vi "UI - FP and Controls.vi"(5 "Term (Methods)":string="Methods", 7 "Msg Chain":string, 8 "error in (no error)":errorcluster {"code" format="Error %.0f"}, 10 "UI Docs":refnum<class "GUI Documentation.lvclass">[](array[class]), 11 "VIDoc Printer - Confluence In":refnum<class "VIDoc Printer - Confluence.lvclass">) -> (0 "error out":errorcluster {"code" format="Error %.0f"}, 3 "VIDoc Printer - Confluence Out":refnum<class "VIDoc Printer - Confluence.lvclass">)   [LabVIEW 2023, in "VIDoc Printer - Confluence.lvlib" / "VIDoc Printer - Confluence.lvclass"]
uses:
  VIDoc Printer - Confluence.lvclass
  C:/projects/DMC/GitHub/DMC CLI VIDoc/Source/Documentation Generation/Printers/Printer/VIDoc Printer.lvclass
  Parsing/GUI Documentation/GUI Documentation.lvclass
  Printer/VIDoc Printer.lvclass/VIDoc Printer.ctl
  Parsing/GUI Documentation/GUI Documentation.lvclass/GUI Documentation.ctl
  VIDoc Printer - Confluence.lvclass/VIDoc Printer - Confluence.ctl
  Confluence Formatting/Types/Format Combo Box.ctl
  Types/VI Info Image Types.ctl
  81eb6c55-aa97-43e1-ad41-127c3d76b8c9.vi
  Printer/Accessors/Get VI Settings - Method Options - Front Panels.vi
  Printer/Accessors/Get VI Settings - Method Options - Options.vi
  Printer/Accessors/Get VI Settings - Method Options - Controls.vi
  Printer/Accessors/Get VI Settings - Controls Detail Level.vi
  Accessors/Get VI Controls Expand.vi
  Accessors/Get Sortable Tables.vi
  Parsing/GUI Documentation/Get VI Info.vi
  Parsing/GUI Documentation/Get Name.vi
  Confluence Formatting/Confluence Formatting.lvlib
  Printer/VIDoc Printer.lvclass
  UI Interaction/UI Interaction.lvclass
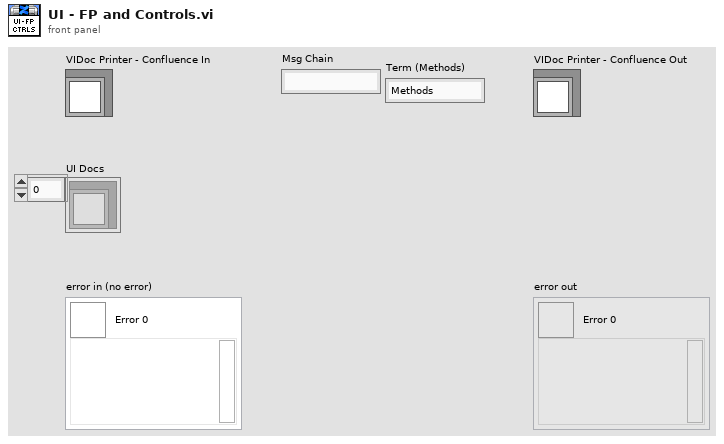
[diagram p1: front panel]
types:
  T1 = typedef "VIDoc Printer.lvlib/Printer Settings.lvclass/VI Settings.ctl" = cluster{"Memory":bool, "By Folder":bool, "By Tree":bool, "By List":bool, "Methods":bool, "Method Options":cluster{"Front Panels":bool, "Options":bool, "Controls":bool}, "List Detail Level":T2, "Methods Detail Level":T2, "Controls Detail Level":T2}
  T2 = typedef "VIDoc Printer.lvlib/Printer Settings.lvclass/Detail Level Enum.ctl" = enum16{"None", "Minimal", "Standard", "Full"}
  T3 = typedef "VIDoc Printer - Confluence.lvlib/VIDoc Printer - Confluence.lvclass/VI Info Image Types.ctl" = enum16{"Conpane", "FP", "BD", "Icon"}
  T4 = typedef "Confluence Formatting.lvlib/Format Combo Box.ctl" = string
  T5 = typedef "VIDoc Parsing.lvlib/Method Spec Cluster.ctl" = cluster{"VI Type Ext":T6, "Name":string, "Path":path, "Get Conpane Image":T7, "Description":string, "Get Library Access Scope":enum32{"invalid scope", "public", "private", "protected", "community"}, "Dispatch":T8, "ContainsCompiledCode":bool, "Exec.IsReentrant":bool, "Exec.ReentrancyType":enum16{"Share clones between instances", "Preallocate clone for each instance"}, "ExecInlining":bool, "ExecInlineIfPossible":bool, "Auto Err Handling":bool, "CodeComplexity":sgl, "Bookmark Tags":string[], "Control VI Type":enum32{"not a control VI", "control", "typedef", "strict typedef"}, "Controls":T9[], "VI Type":enum32{"invalid VI type", "Standard VI", "Control VI", "Global VI", "Polymorphic VI", "Configuration VI", "SubSystem", "Facade VI", "Method VI", "Statechart Diagram VI"}, "Minimum Size":T11, "Front Panel Window:Title":string, "Front Panel Window:Behavior":enum32{"Invalid", "Default", "Floating", "Floating/Auto-Hide", "Modal"}, "Front Panel Window:Closeable":bool, "Must Override":bool, "Must Use Parent Implementation":bool, "VI Icon":T7, "Front Panel":T7, "History:Revision Number":u32, "Metrics:Total Data Size":u32, "Execution:Allow Debugging":bool, "Execution:Preferred Exec System":enum32{"invalid execution system", "user interface", "standard", "instrument i/o", "data acquisition", "other 1", "other 2", "same as caller"}, "Execution:Priority":enum32{"invalid priority", "background priority", "normal priority", "above normal priority", "high priority", "time critical priority", "subroutine"}, "BM Tag Text":string[], "Block Diagram":T7, "Structure Tree":T12[]}
  T6 = typedef "VIDoc Parsing.lvlib/VI Type Extended Enum.ctl" = enum16{"Unknown", "Class Method", "Class Accessor Get", "Class Accessor Set", "Class Control", "Library Method", "Library Control", "VI", "Control"}
  T7 = typedef "imagedata.ctl" = cluster{"image type":i32, "image depth":i32, "image":u8[], "mask":u8[], "colors":u32[], "Rectangle":cluster{"left":i16, "top":i16, "right":i16, "bottom":i16}}
  T8 = typedef "VIDoc Parsing.lvlib/Class Dispatch Type Enum.ctl" = enum16{"None", "Static", "Dynamic"}
  T9 = typedef "VIDoc Parsing.lvlib/Controls Info Cluster.ctl" = cluster{"Name":string, "Description":string, "Data Type":string, "Tip Strip":string, "UID":i32, "Image Data":T7, "ToggleKeyBind":T10, "Raw Label":string, "Raw Caption":string}
  T10 = typedef "LVKeyTypeDef.ctl" = cluster{"Focus":bool, "Control":bool, "Shift":bool, "Key":string}
  T11 = typedef "LVPointTypeDef.ctl" = cluster{"Horizontal":i16, "Vertical":i16}
  T12 = typedef "VIDoc Parsing.lvlib/Structure Reporter.lvlib/Tree Cluster.ctl" = cluster{"Object Class Name":string, "Labels":string[], "Child Tag":string, "Item Indent":i32, "Child Only?":bool, "Glyph Index":i32}
  T13 = enum32{"not a control VI", "control", "typedef", "strict typedef"}
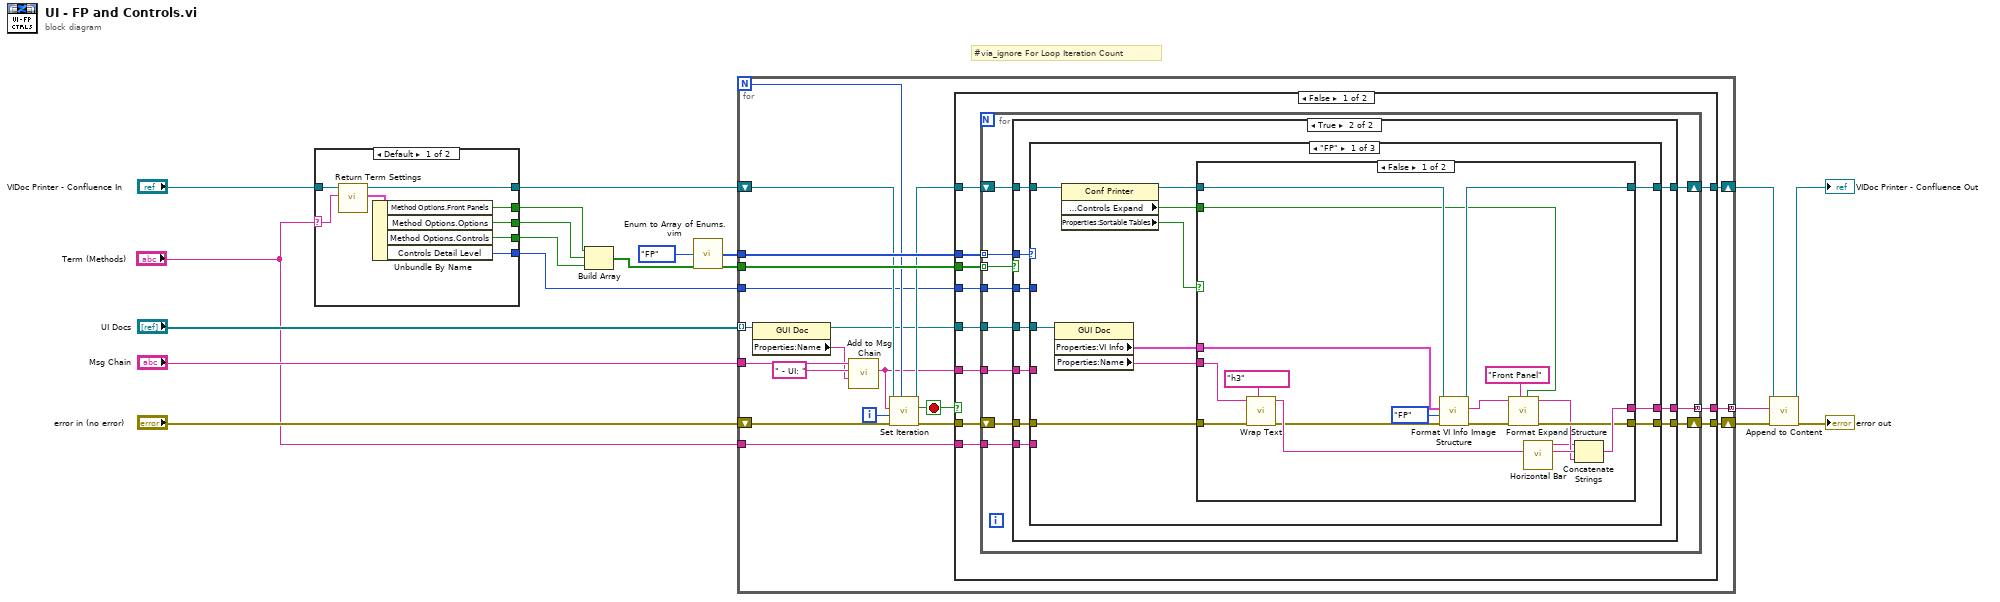
[diagram p0: block diagram]
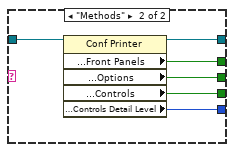
[diagram p2: hidden frame]
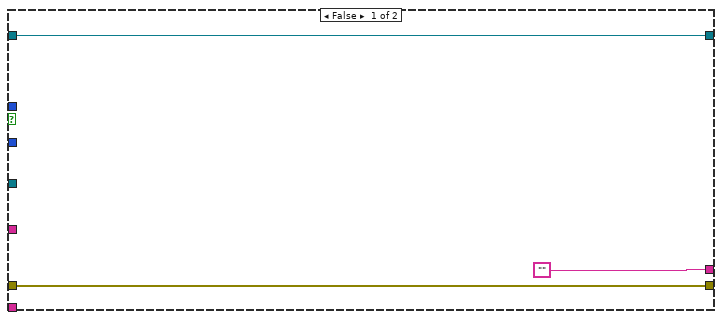
[diagram p3: hidden frame]
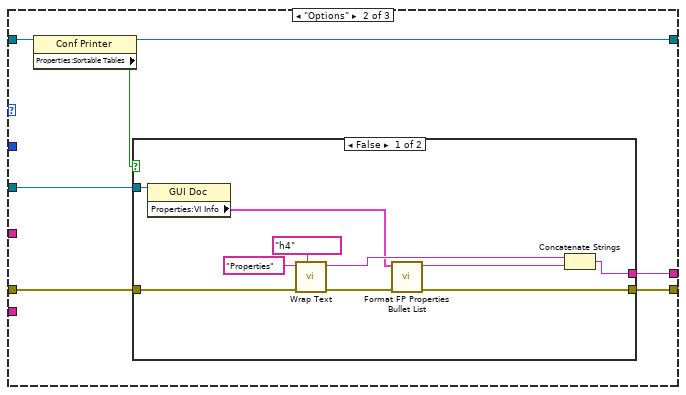
[diagram p5: hidden frame]
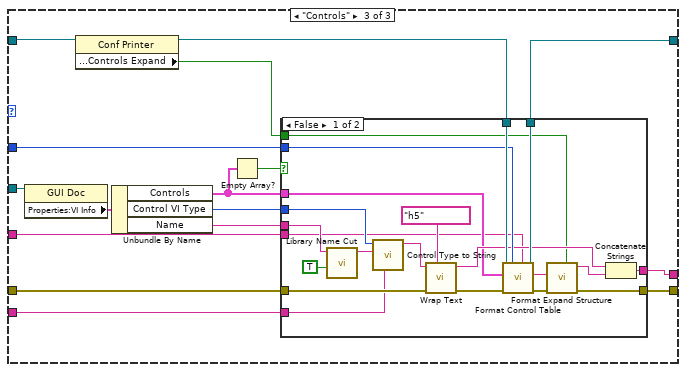
[diagram p7: hidden frame]
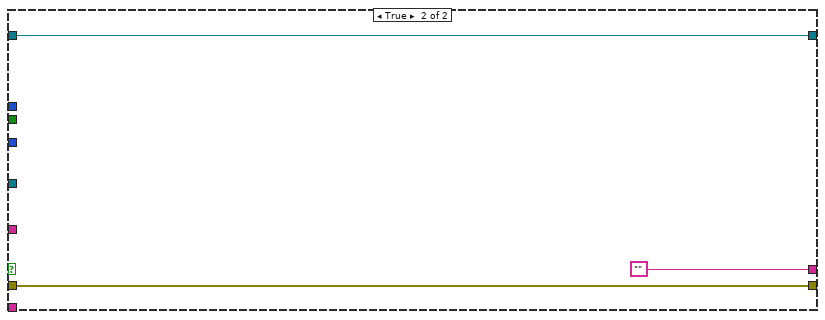
[diagram p9: hidden frame]
diagram:
  # "#via_ignore For Loop Iteration Count"
  n1 = case shown="Default" "Term (Methods)" {
    selector: "Term (Methods)" -> [w24 _]
    tunnel: "VIDoc Printer - Confluence In" -> [w26 w32]
    tunnel: [w25 w31] -> w9
    tunnel: [w22 w30] -> w5
    tunnel: [w21 w29] -> w4
    tunnel: [w20 w28] -> w3
    tunnel: [w19 w27] -> w2
    frame Default {
      n2 = call "Return Term Settings.vi"("Term"=w24, "Printer in"=w26) -> ("Term Settings"=w23:T1, "Printer out"=w25:refnum<class "VIDoc Printer - Confluence.lvclass">)  [unwired: 6 in, 2 out]
      n3 = Unbundle By Name(w23) -> ("Method Options.Front Panels"=w22:bool, "Method Options.Options"=w21:bool, "Method Options.Controls"=w20:bool, "Controls Detail Level"=w19:T2)
    }
    frame "Methods" {
      n4 = property class="Conf Printer"(reference=w32) -> (reference out=w31:refnum<class "VIDoc Printer - Confluence.lvclass">, "Properties:Settings:VI Members:Front Panels"=w30:bool, "Properties:Settings:VI Members:Options"=w29:bool, "Properties:Settings:VI Members:Controls"=w28:bool, "Properties:Settings:VI Members:Controls Detail Level"=w27:T2)  [unwired: 1 in, 1 out]
    }
  }
  n5 = Build Array(w5, w4, w3) -> (w6:bool[])
  n6 = call "Enum to Array of Enums.vim"("enum"=enum16{"FP", "Options", "Controls"}."FP") -> ("array of enums"=w7:enum16{"FP", "Options", "Controls"}[])
  n7 = for {
    N -> [w43]
    shift-right: [w51] -> w13
    shift-left: "error in (no error)" -> [w45]
    shift-right: [w52] -> w16
    shift-left: w9 -> [w47]
    tunnel: "UI Docs" -> [w50] mode=indexing
    tunnel: w7 -> [w49]
    tunnel: w6 -> [w48]
    tunnel: "Msg Chain" -> [w40]
    tunnel: [w36] -> w12 mode=concatenating
    tunnel: "Term (Methods)" -> [w35]
    tunnel: w2 -> [w34]
    i -> [w42]
    stop <- w37 stop-if-true
    n8 = property class="GUI Doc"(reference=w50) -> (reference out=w39:refnum<class "GUI Documentation.lvclass">, "Properties:Name"=w38:string)  [unwired: 1 in, 1 out]
    n9 = call "Add to Msg Chain.vi"("New"=w38, "Separator (-)"=" - UI: ", "Msg Chain in"=w40) -> ("Msg Chain out"=w33:string)  [unwired: 8 in]
    n10 = call "Set Iteration.vi"("Progress Max"=w43, "error in (no error)"=w45, "Progress Value"=w42, "Message (No Message Update)"=w33, "VIDoc Printer In"=w47) -> ("error out"=w44:errorcluster, "Abort?"=w37:bool, "VIDoc Printer Out"=w46:refnum<class "VIDoc Printer - Confluence.lvclass">)  [unwired: 4 in]
    n11 = case shown="False" w37 {
      tunnel: [w63 w177] -> w52
      tunnel: [w62 w176] -> w51
      tunnel: w49 -> [w61 _]
      tunnel: w48 -> [w60 _]
      tunnel: w46 -> [w59 w177]
      tunnel: w44 -> [w58 w176]
      tunnel: w39 -> [w57 _]
      tunnel: [w56 ""] -> w36
      tunnel: w35 -> [w55 _]
      tunnel: w34 -> [w54 _]
      tunnel: w33 -> [w53 _]
      frame False {
        n12 = for {
          shift-right: [w73] -> w63
          shift-left: w59 -> [w72]
          shift-right: [w71] -> w62
          shift-left: w58 -> [w70]
          tunnel: w57 -> [w68]
          tunnel: w61 -> [w69] mode=indexing
          tunnel: w60 -> [w74] mode=indexing
          tunnel: [w67] -> w56 mode=concatenating
          tunnel: w55 -> [w66]
          tunnel: w54 -> [w65]
          tunnel: w53 -> [w64]
          n13 = case shown="True" w74 {
            tunnel: [w77 w82] -> w73
            tunnel: w72 -> [w77 w83]
            tunnel: [w76 w84] -> w71
            tunnel: w70 -> [w76 w86]
            tunnel: w69 -> [_ w87]
            tunnel: w68 -> [_ w85]
            tunnel: ["" w81] -> w67
            tunnel: w66 -> [_ w80]
            tunnel: w65 -> [_ w79]
            tunnel: w64 -> [_ w78]
            frame False {
            }
            frame True {
              n14 = case shown="\"FP\"" w87 {
                tunnel: w86 -> [w95 w122 w146]
                tunnel: w85 -> [w96 w124 w148]
                tunnel: [w91 w120 w150] -> w84
                tunnel: w83 -> [w94 w121 w151]
                tunnel: [w93 w119 w149] -> w82
                tunnel: [w92 w123 w141] -> w81
                tunnel: w80 -> [_ _ w145]
                tunnel: w79 -> [_ _ w147]
                tunnel: w78 -> [_ _ w136]
                frame "FP" {
                  n15 = property class="GUI Doc"(reference=w96) -> ("Properties:VI Info"=w98:T5, "Properties:Name"=w97:string)  [unwired: 1 in, 2 out]
                  n16 = property class="Conf Printer"(reference=w94) -> (reference out=w90:refnum<class "VIDoc Printer - Confluence.lvclass">, "Properties:Expand?:VI:Controls Expand"=w89:bool, "Properties:Sortable Tables"=w88:bool)  [unwired: 1 in, 1 out]
                  n17 = case shown="False" w88 {
                    tunnel: w98 -> [w101 _]
                    tunnel: w97 -> [w115 _]
                    tunnel: w95 -> [w112 w116]
                    tunnel: [w111 w117] -> w93
                    tunnel: [w110 _] -> w92
                    tunnel: [w108 w116] -> w91
                    tunnel: w90 -> [w103 w117]
                    tunnel: w89 -> [w102 _]
                    frame False {
                      n18 = call "Wrap Text.vi"("Formatting"=T4 "h3", "Error in"=w112, "String"=w115) -> ("Error out"=w99:errorcluster, "Wrapped String"=w114:string)  [unwired: 7 in]
                      n19 = call "Format VI Info Image Structure.vi"("Error in"=w99, "Image Type"=VI_Info_Image_Types."FP", "VI Info"=w101, "VIDoc Printer - Confluence In"=w103) -> ("Error out"=w109:errorcluster, "Image Structure Text"=w106:string, "VIDoc Printer - Confluence Out"=w111:refnum<class "VIDoc Printer - Confluence.lvclass">)  [unwired: 4 in, 1 out]
                      n20 = call "Format Expand Structure.vi"("Enable? (T)"=w102, "Title (Click here to expand...)"="Front Panel" ("String"), "Error in"=w109, "Content"=w106) -> ("Error out"=w108:errorcluster, "Expand String"=w105:string)  [unwired: 6 in]
                      n21 = call "Horizontal Bar.vi"() -> ("Horizontal Bar"=w104:string)  [unwired: 11 in]
                      n22 = Concatenate Strings(w104, w114, w105) -> (w110:string)
                    }
                    frame True {
                      # "Sortable Tables Contains FP"
                    }
                  }
                }
                frame "Options" {
                  n23 = property class="Conf Printer"(reference=w121) -> (reference out=w119:refnum<class "VIDoc Printer - Confluence.lvclass">, "Properties:Sortable Tables"=w118:bool)  [unwired: 1 in, 1 out]
                  n24 = case shown="False" w118 {
                    tunnel: w124 -> [w131 _]
                    tunnel: [w130 _] -> w123
                    tunnel: w122 -> [w129 w135]
                    tunnel: [w125 w135] -> w120
                    frame False {
                      n25 = property class="GUI Doc"(reference=w131) -> ("Properties:VI Info"=w128:T5)  [unwired: 1 in, 2 out]
                      n26 = call "Wrap Text.vi"("Formatting"=T4 "h4", "Error in"=w129, "String"="Properties") -> ("Error out"=w127:errorcluster, "Wrapped String"=w134:string)  [unwired: 7 in]
                      n27 = call "Format FP Properties Bullet List.vi"("Error in"=w127, "VI Info"=w128) -> ("Error out"=w125:errorcluster, "FP Properties Bullets"=w126:string)  [unwired: 8 in]
                      n28 = Concatenate Strings(w134, w126) -> (w130:string)
                    }
                    frame True {
                      # "Displayed in Table"
                    }
                  }
                }
                frame "Controls" {
                  n29 = property class="GUI Doc"(reference=w148) -> ("Properties:VI Info"=w144:T5)  [unwired: 1 in, 2 out]
                  n30 = property class="Conf Printer"(reference=w151) -> (reference out=w138:refnum<class "VIDoc Printer - Confluence.lvclass">, "Properties:Expand?:VI:Controls Expand"=w137:bool)  [unwired: 1 in, 1 out]
                  n31 = Unbundle By Name(w144) -> ("Controls"=w140:T9[], "Control VI Type"=w142:T13, "Name"=w143:string)
                  n32 = Empty Array?(array=w140) -> (empty?=w139:bool)
                  n33 = case shown="False" w139 {
                    tunnel: w138 -> [w172 w173]
                    tunnel: [w156 w174] -> w150
                    tunnel: [w170 w173] -> w149
                    tunnel: w147 -> [w169 _]
                    tunnel: w146 -> [w165 w174]
                    tunnel: w145 -> [w163 _]
                    tunnel: w143 -> [w162 _]
                    tunnel: w142 -> [w161 _]
                    tunnel: [w160 _] -> w141
                    tunnel: w140 -> [w158 _]
                    tunnel: w137 -> [w153 _]
                    tunnel: w136 -> [w152 _]
                    frame False {
                      n34 = call "Library Name Cut.vi"("Cut? (T)"=TRUE ("Cut?"), "Name in"=w162) -> ("Name out"=w168:string)  [unwired: 9 in]
                      n35 = call "Control Type to String.vi"("Term (Methods)"=w163, "Lib Name"=w168, "Control VI Type"=w161) -> ("String"=w167:string)  [unwired: 8 in]
                      n36 = call "Wrap Text.vi"("Formatting"=T4 "h5", "Error in"=w165, "String"=w167) -> ("Error out"=w164:errorcluster, "Wrapped String"=w159:string)  [unwired: 7 in]
                      n37 = call "Format Control Table.vi"("Msg Chain in"=w152, "Controls Opt"=w169, "error in (no error)"=w164, "Controls"=w158, "VIDoc Printer - Confluence In"=w172) -> ("error out"=w171:errorcluster, "Table"=w155:string, "VIDoc Printer - Confluence Out"=w170:refnum<class "VIDoc Printer - Confluence.lvclass">)  [unwired: 4 in]
                      n38 = call "Format Expand Structure.vi"("Enable? (T)"=w153, "Error in"=w171, "Content"=w155) -> ("Error out"=w156:errorcluster, "Expand String"=w154:string)  [unwired: 7 in]
                      n39 = Concatenate Strings(w159, w154) -> (w160:string)
                    }
                    frame True {
                    }
                  }
                }
              }
            }
          }
        }
      }
      frame True {
      }
    }
  }
  n40 = call "Append to Content.vi"("error in (no error)"=w13, "Content"=w12, "VIDoc Printer - Confluence In"=w16) -> ("error out"=→"error out":errorcluster, "VIDoc Printer - Confluence Out"=→"VIDoc Printer - Confluence Out":refnum<class "VIDoc Printer - Confluence.lvclass">)  [unwired: 7 in]
